vi "Result.Test Result to Factory Logix Xlink Adapter.vi"(5 "Overall Result Only":bool, 6 "Prefixes":T1={"Test Run"="TestRun.", "Client Setup"="StaSetup.", "Client SW"="StaSW.", "Client HW"="StaHW.", "Attribute"="Str.", "Numeric"="Num.", "Client ID"="Sta."}, 7 "Remove Headings":bool, 8 "error in":errorcluster, 9 "Add Prefixes":bool, 10 "Test Result":T2={"#attributes"={"Version"="MTE_1.0.0"}, "Station"={"Name"="", "PN"="", "SN"="", "Rev"="", "PC Name"="", "Location"="", "HW_Config"={"HW_Item"=[]}, "SW_Config"={"SW_Item"=[]}}, "Test Run"={"Operator"="", "Start Time"=timestamp(0 s since 1904-01-01), "Duration(s)"=0.0, "Mode"="", "Comment"="", "ProcessStep"=""}, "Test Sequence"={"Name"="", "Config"={"Config_Item"=[]}}, "UUTs"={"UUT"=[]}} {"UUTs"."UUT"."Measurements"."Measurement"."Status" items=["LOG", "PASS", "FAIL", "ERROR"]}, 11 "Path":path) -> (0 "error out":errorcluster)   [LabVIEW 2018]
uses:
  TestResult.FullResultData.ctl
  TestResult.Station Info.ctl
  TestResult.HW Item.ctl
  TestResult.SW Item.ctl
  TestResult.Test Run Info.ctl
  TestResult.Test Info.ctl
  TestResult.UUT Result.ctl
  TestResult.Symptom.ctl
  TestResult.Symptom.State.ctl
  Result.Measurement Item.ctl
  Result.Measurement and Attribute Item Status.ctl
  TestResult.UUTInfo.ctl
  Result.Factory Logix XLink Adapter, Data Prefixes.ctl
  Result.Factory Logix XLink Adapter, Measurement Item.ctl
  Result.Factory Logix XLink Adapter.ctl
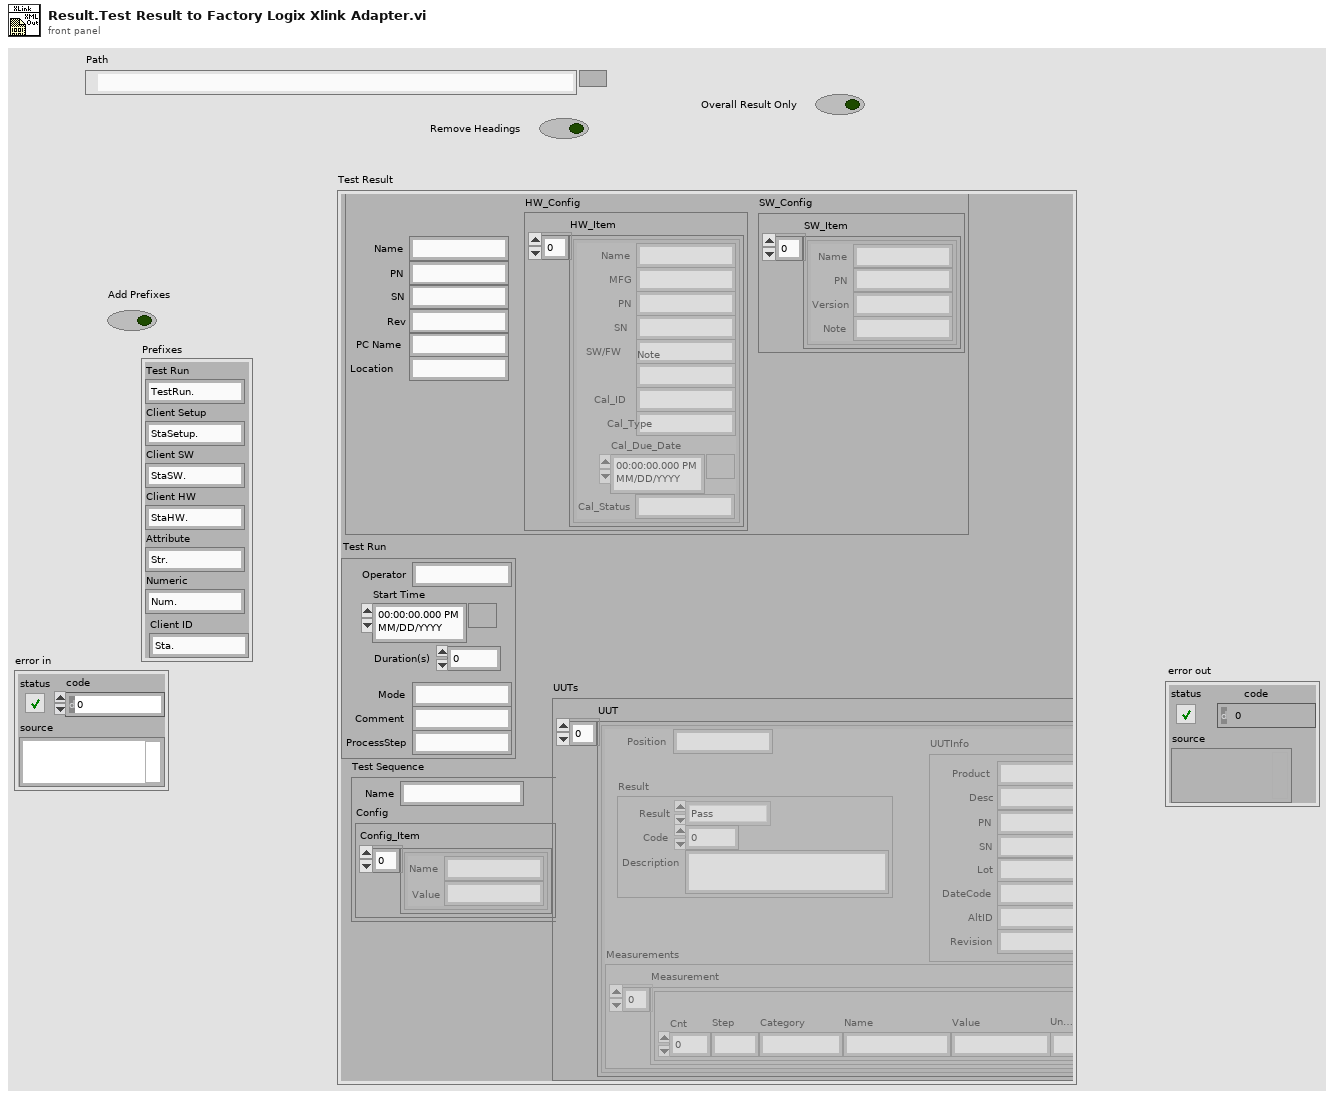
[diagram p1: front panel]
types:
  T1 = typedef "Result.Factory Logix XLink Adapter, Data Prefixes.ctl" = cluster{"Test Run":string, "Client Setup":string, "Client SW":string, "Client HW":string, "Attribute":string, "Numeric":string, "Client ID":string}
  T2 = typedef "TestResult.FullResultData.ctl" = cluster{"#attributes":cluster{"Version":string}, "Station":T3, "Test Run":T6, "Test Sequence":T7, "UUTs":cluster{"UUT":T8[]}}
  T3 = typedef "TestResult.Station Info.ctl" = cluster{"Name":string, "PN":string, "SN":string, "Rev":string, "PC Name":string, "Location":string, "HW_Config":cluster{"HW_Item":T4[]}, "SW_Config":cluster{"SW_Item":T5[]}}
  T4 = typedef "TestResult.HW Item.ctl" = cluster{"Name":string, "MFG":string, "PN":string, "SN":string, "SW/FW":string, "Note":string, "Cal_ID":string, "Cal_Type":string, "Cal_Due_Date":timestamp, "Cal_Status":string}
  T5 = typedef "TestResult.SW Item.ctl" = cluster{"Name":string, "PN":string, "Version":string, "Note":string}
  T6 = typedef "TestResult.Test Run Info.ctl" = cluster{"Operator":string, "Start Time":timestamp, "Duration(s)":dbl, "Mode":string, "Comment":string, "ProcessStep":string}
  T7 = typedef "TestResult.Test Info.ctl" = cluster{"Name":string, "Config":cluster{"Config_Item":cluster{"Name":string, "Value":string}[]}}
  T8 = typedef "TestResult.UUT Result.ctl" = cluster{"Position":string, "Result":T9, "Measurements":cluster{"Measurement":T11[]}, "UUTInfo":T13}
  T9 = typedef "TestResult.Symptom.ctl" = cluster{"Result":T10, "Code":i32, "Description":string}
  T10 = typedef "TestResult.Symptom.State.ctl" = enum16{"Pass", "Fail", "Error", "Aborted", "Completed", "Logged"}
  T11 = typedef "Result.Measurement Item.ctl" = cluster{"Cnt":i32, "Step":string, "Category":string, "Name":string, "Value":string, "Units":string, "LimType":string, "LL":string, "UL":string, "Status":T12, "Code":i32, "Desc":string, "Time":timestamp}
  T12 = typedef "Result.Measurement and Attribute Item Status.ctl" = i32
  T13 = typedef "TestResult.UUTInfo.ctl" = cluster{"Product":string, "Desc":string, "PN":string, "SN":string, "Lot":string, "DateCode":string, "AltID":string, "Revision":string, "Properties":cluster{"Property":cluster{"Name":string, "Value":string}[]}}
  T14 = typedef "Result.Factory Logix XLink Adapter, Measurement Item.ctl" = cluster{"Name":string, "Sequence":i32, "Measurement Type":string, "Result":string, "Value":string, "Units":string, "Nominal":string, "LowerLimit":string, "UpperLimit":string, "FailDesc":string, "DateAndTime":string}
  T15 = typedef "Result.Factory Logix XLink Adapter.ctl" = cluster{"Operator":string, "ParentBarcode":string, "Measurements":cluster{"Measurement":T14[]}}
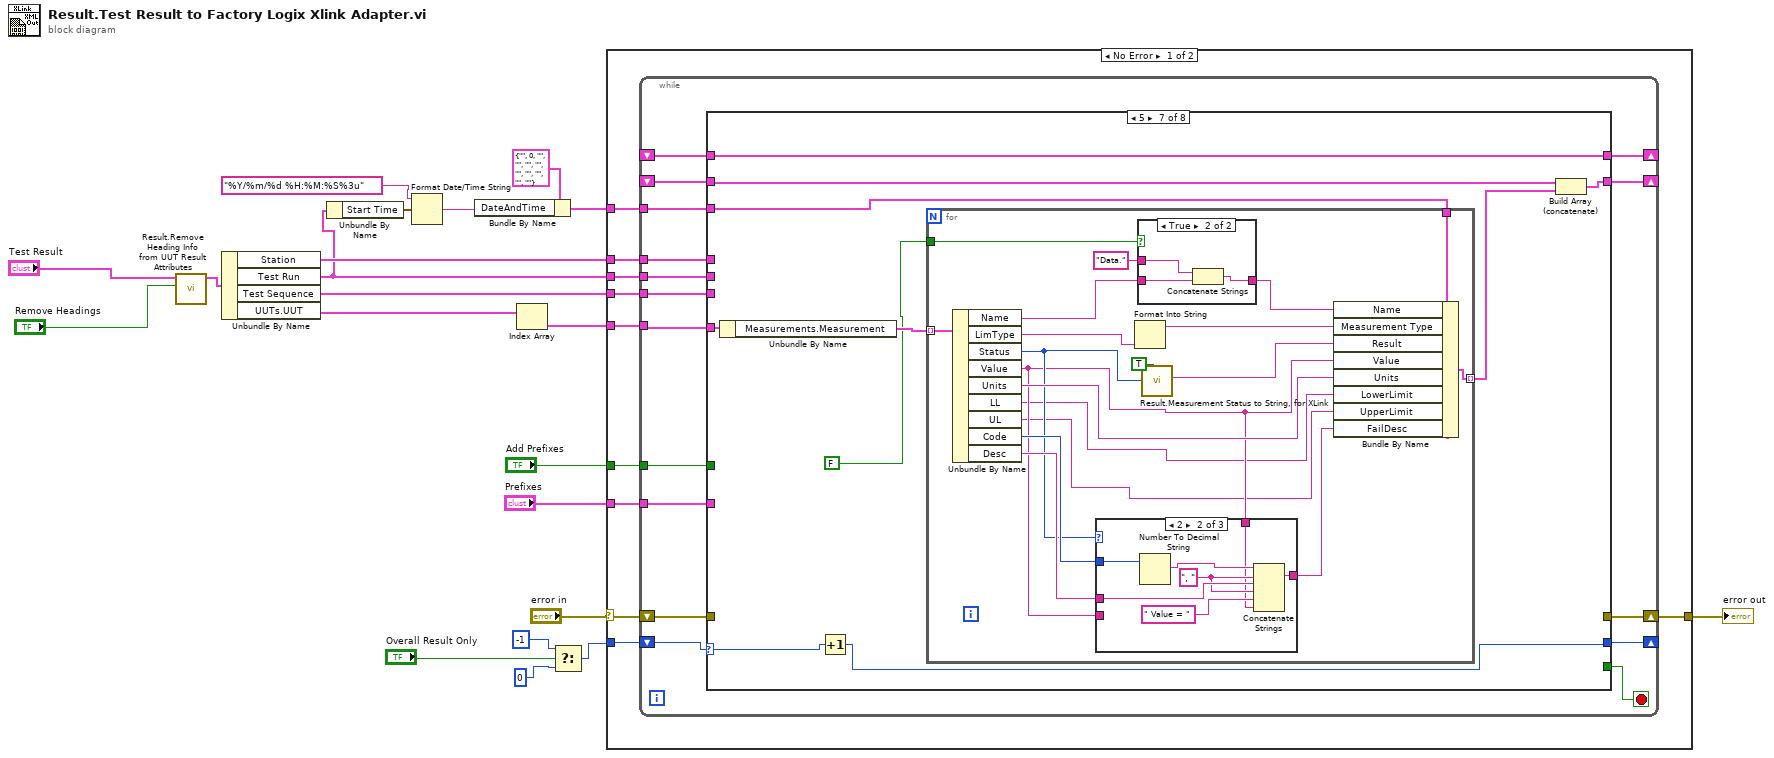
[diagram p0: block diagram]
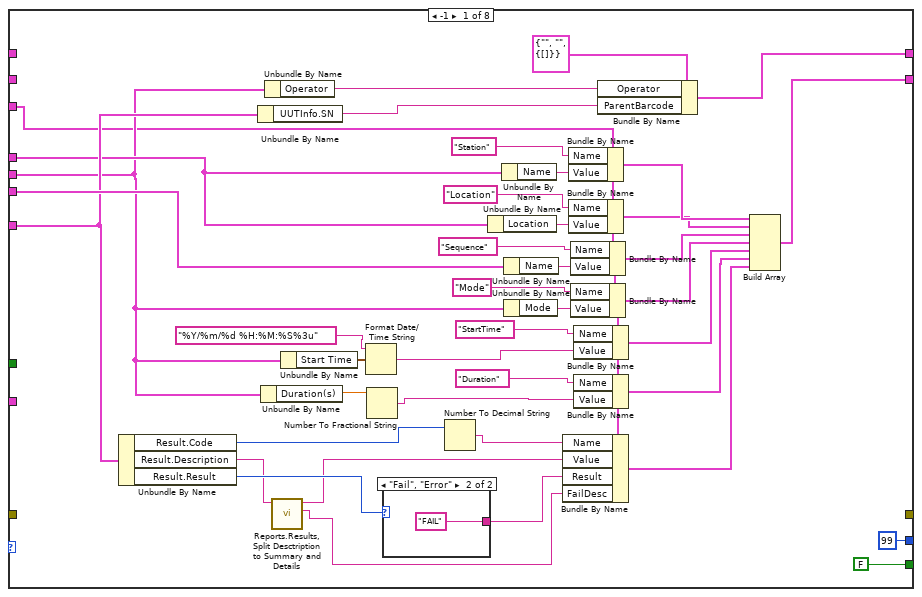
[diagram p2: hidden frame]
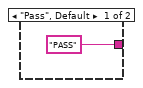
[diagram p3: hidden frame]
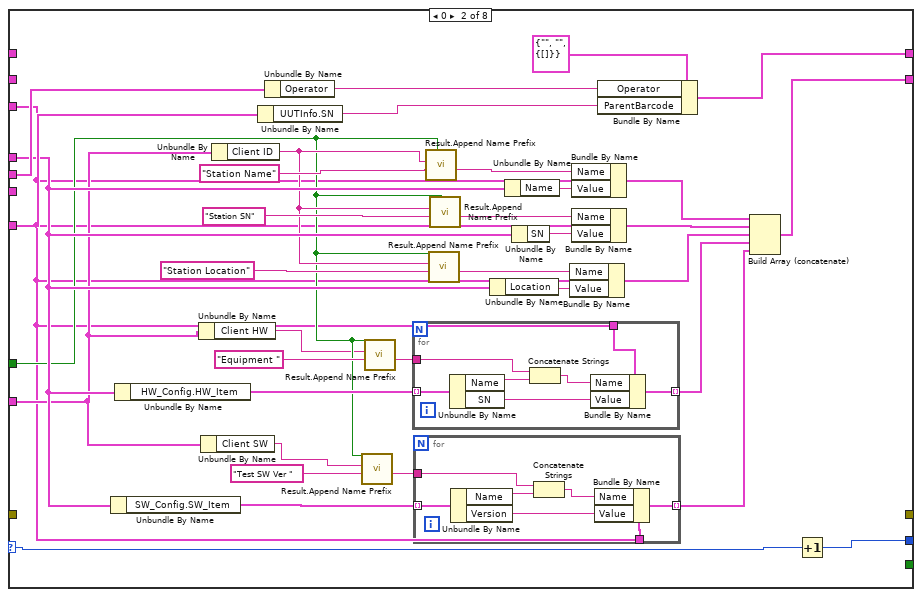
[diagram p4: hidden frame]
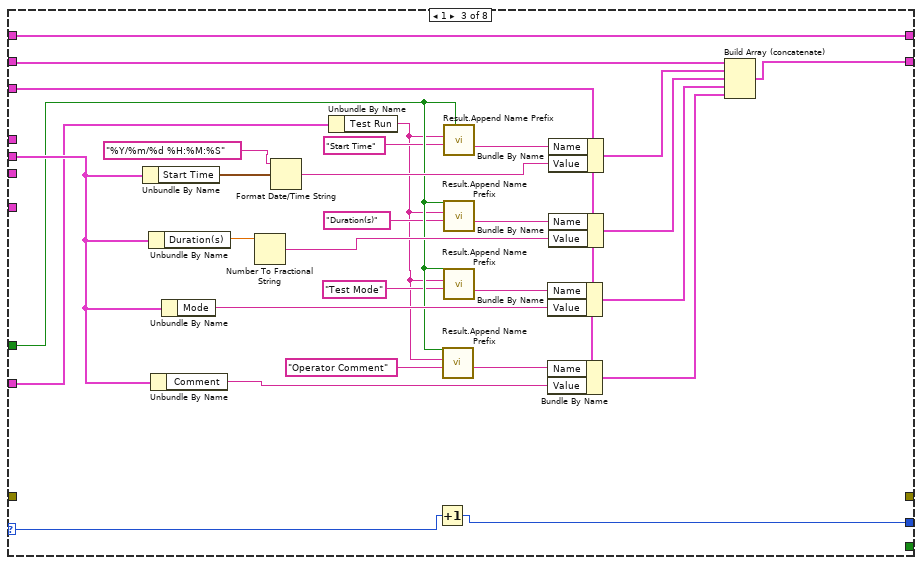
[diagram p5: hidden frame]
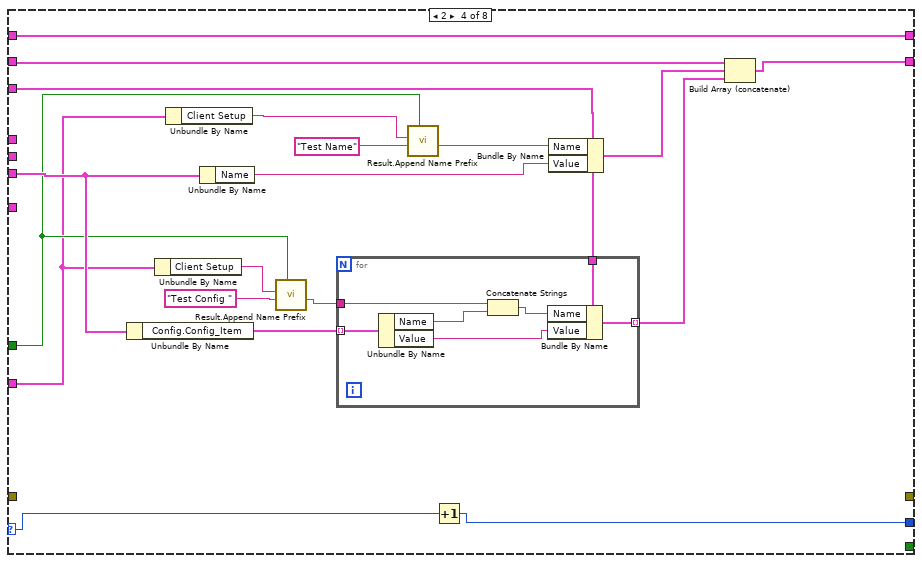
[diagram p6: hidden frame]
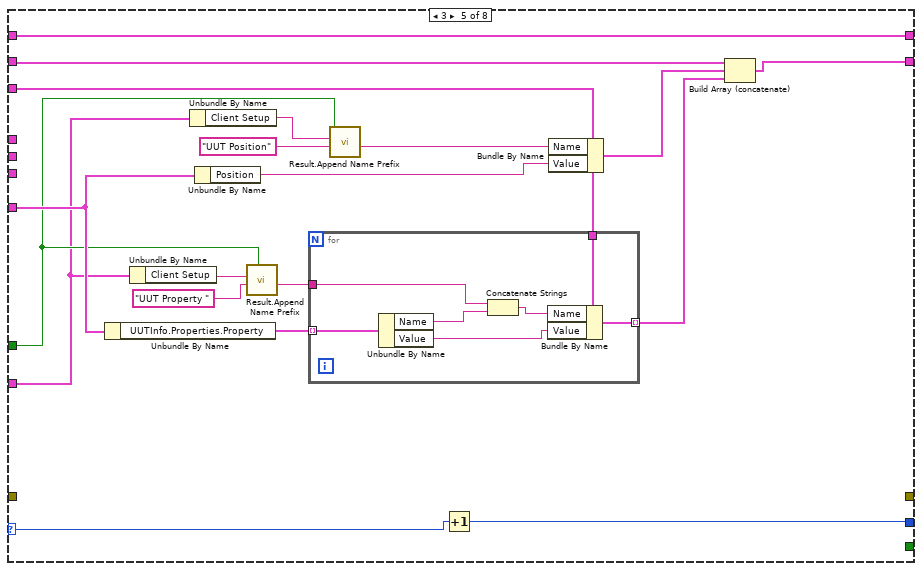
[diagram p7: hidden frame]
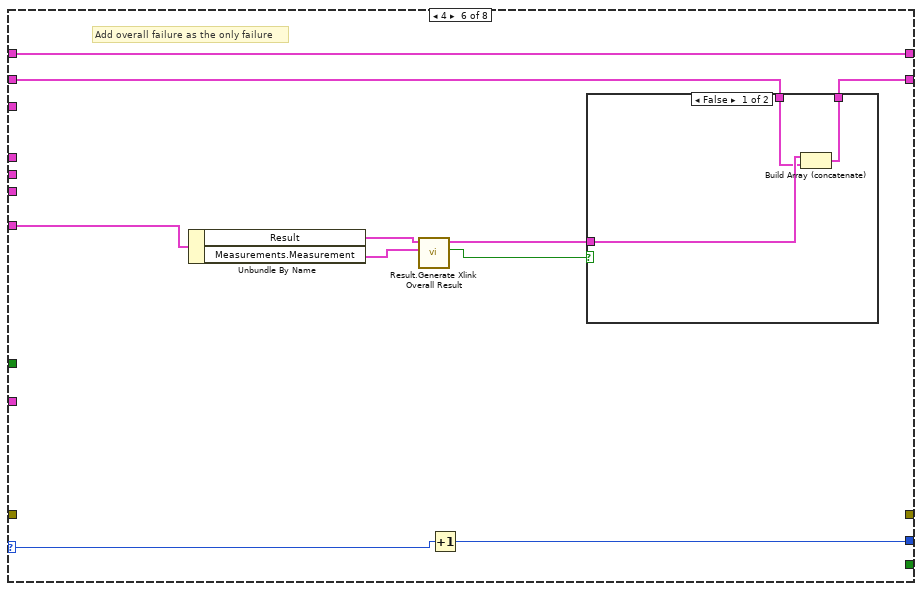
[diagram p8: hidden frame]
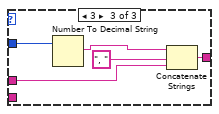
[diagram p12: hidden frame]
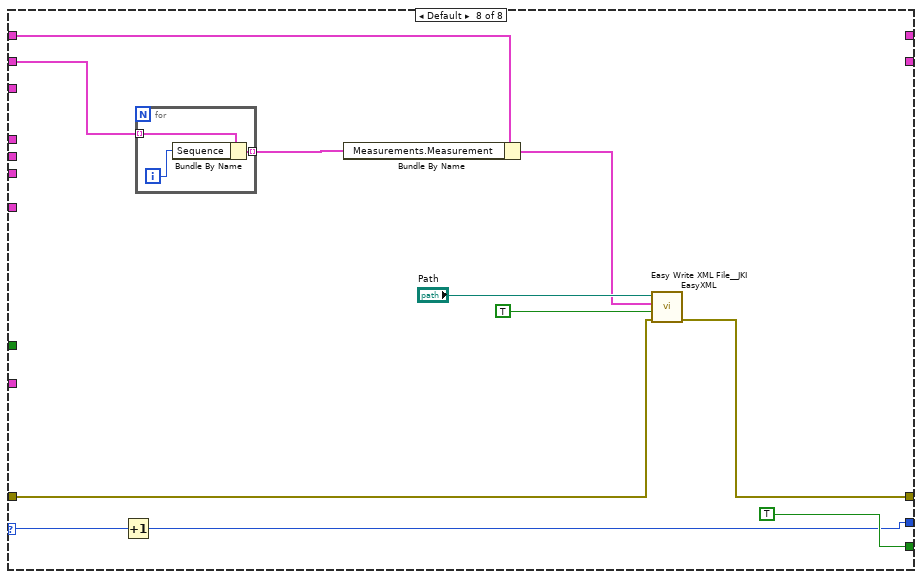
[diagram p13: hidden frame]
diagram:
  n1 = call "Result.Remove Heading Info from UUT Result Attributes.vi"("Remove Headings"="Remove Headings", "Data"="Test Result") -> ("Data Out"=w14:T2)  [unwired: 9 in]
  n2 = Unbundle By Name(w14) -> ("Station"=w17:T3, "Test Run"=w6:T6, "Test Sequence"=w16:T7, "UUTs.UUT"=w19:T8[])
  n3 = Unbundle By Name(w6) -> ("Start Time"=w7:timestamp)
  n4 = Format Date/Time String(time format string (%c)="%Y/%m/%d %H:%M:%S%3u", seconds (now)=w7) -> (date/time string=w5:string)  [unwired: 1 in]
  n5 = Bundle By Name(cluster=T14 {"Name"="", "Sequence"=0, "Measurement Type"="", "Result"="", "Value"="", "Units"="", "Nominal"="", "LowerLimit"="", "UpperLimit"="", "FailDesc"="", "DateAndTime"=""} ("Measurement"), "DateAndTime"=w5) -> (w9:T14)
  n6 = Index Array(array=w19) -> (element=w18:T8)  [unwired: 1 in]
  n7 = Select(t=-1, s="Overall Result Only", f=0) -> (s? t:f=w1:i32)
  n8 = case shown="No Error" "error in" {
    selector: "error in" -> [w30 w295]
    tunnel: [w31 w295] -> w21
    tunnel: w18 -> [w29 _]
    tunnel: w17 -> [w28 _]
    tunnel: w6 -> [w27 _]
    tunnel: w16 -> [w26 _]
    tunnel: "Prefixes" -> [w25 _]
    tunnel: "Add Prefixes" -> [w24 _]
    tunnel: w9 -> [w23 _]
    tunnel: w1 -> [w22 _]
    frame No Error {
      n9 = while {
        shift-right: [w47] -> w31
        shift-left: w30 -> [w46]
        shift-right: [w44] -> _
        shift-left: _ -> [w45]
        tunnel: w29 -> [w42]
        tunnel: w28 -> [w40]
        tunnel: w27 -> [w43]
        tunnel: w26 -> [w39]
        shift-right: [w41] -> _
        shift-left: _ -> [w37]
        tunnel: w25 -> [w36]
        tunnel: w24 -> [w35]
        tunnel: w23 -> [w34]
        shift-right: [w32] -> _
        shift-left: w22 -> [w33]
        stop <- w38 stop-if-true
        n10 = case shown="5" w33 {
          selector: w33 -> [_ w91 w142 w171 w197 w223 w237 w282]
          tunnel: [_ _ _ _ _ _ _ w290] -> w47
          tunnel: w46 -> [_ _ _ _ _ _ _ w288]
          tunnel: w45 -> [_ _ w169 w188 w214 w231 w245 w287]
          tunnel: [w87 w125 w169 w188 w214 w231 w245 _] -> w44
          tunnel: w43 -> [w55 w124 w162 _ _ _ _ _]
          tunnel: w42 -> [w74 w123 _ _ w207 w228 w241 _]
          tunnel: [w83 w119 w166 w185 w211 w229 w240 _] -> w41
          tunnel: w37 -> [_ _ w168 w187 w213 w230 w244 w286]
          tunnel: w40 -> [w66 w109 _ _ _ _ _ _]
          tunnel: w39 -> [w75 _ _ w184 _ _ _ _]
          tunnel: [FALSE _ _ _ _ _ _ TRUE] -> w38
          tunnel: w36 -> [_ w96 w145 w174 w199 _ _ _]
          tunnel: w35 -> [_ w97 w154 w176 w202 _ _ _]
          tunnel: w34 -> [w53 w93 w143 w172 w198 _ w238 _]
          tunnel: [99 w92 w141 w170 w196 w222 w236 w281] -> w32
          frame -1 {
            n11 = Unbundle By Name(w74) -> ("Result.Code"=w73:i32, "Result.Description"=w50:string, "Result.Result"=w71:T10)
            n12 = Unbundle By Name(w74) -> ("UUTInfo.SN"=w86:string)
            n13 = Unbundle By Name(w55) -> ("Duration(s)"=w56:dbl)
            n14 = Unbundle By Name(w55) -> ("Operator"=w85:string)
            n15 = call "Reports.Results, Split Desctription to Summary and Details.vi"("Description"=w50) -> ("Details"=w48:string, "Summary Description"=w49:string)  [unwired: 9 in]
            n16 = Unbundle By Name(w55) -> ("Start Time"=w59:timestamp)
            n17 = Format Date/Time String(time format string (%c)="%Y/%m/%d %H:%M:%S%3u", seconds (now)=w59) -> (date/time string=w57:string)  [unwired: 1 in]
            n18 = Number To Fractional String(number=w56) -> (F-format string=w54:string)  [unwired: 3 in]
            n19 = case shown="\"Fail\", \"Error\"" w71 {
              tunnel: ["PASS" "FAIL"] -> w70
              frame "Pass", Default {
              }
              frame "Fail", "Error" {
              }
            }
            n20 = Number To Decimal String(number=w73) -> (decimal integer string=w72:string)  [unwired: 1 in]
            n21 = Unbundle By Name(w66) -> ("Location"=w67:string)
            n22 = Unbundle By Name(w66) -> ("Name"=w82:string)
            n23 = Unbundle By Name(w75) -> ("Name"=w80:string)
            n24 = Unbundle By Name(w55) -> ("Mode"=w77:string)
            n25 = Bundle By Name(cluster=w53, "Name"=w72, "Value"=w49, "Result"=w70, "FailDesc"=w48) -> (w52:T14)
            n26 = Bundle By Name(cluster=w53, "Name"="Station", "Value"=w82) -> (w84:T14)
            n27 = Bundle By Name(cluster=w53, "Name"="Location", "Value"=w67) -> (w65:T14)
            n28 = Bundle By Name(cluster=w53, "Name"="Sequence", "Value"=w80) -> (w79:T14)
            n29 = Bundle By Name(cluster=w53, "Name"="Mode", "Value"=w77) -> (w69:T14)
            n30 = Bundle By Name(cluster=w53, "Name"="StartTime", "Value"=w57) -> (w61:T14)
            n31 = Bundle By Name(cluster=w53, "Name"="Duration", "Value"=w54) -> (w51:T14)
            n32 = Bundle By Name(cluster=T15 {"Operator"="", "ParentBarcode"="", "Measurements"={"Measurement"=[]}} ("TestData"), "Operator"=w85, "ParentBarcode"=w86) -> (w87:T15)
            n33 = Build Array(w84, w65, w79, w69, w61, w51, w52) -> (w83:T14[])
          }
          frame 0 {
            n34 = Unbundle By Name(w109) -> ("SW_Config.SW_Item"=w111:T5[])
            n35 = Unbundle By Name(w109) -> ("HW_Config.HW_Item"=w113:T4[])
            n36 = Unbundle By Name(w96) -> ("Client HW"=w95:string)
            n37 = Unbundle By Name(w96) -> ("Client SW"=w94:string)
            n38 = Unbundle By Name(w96) -> ("Client ID"=w104:string)
            n39 = Unbundle By Name(w123) -> ("UUTInfo.SN"=w122:string)
            n40 = Unbundle By Name(w124) -> ("Operator"=w121:string)
            n41 = call "Result.Append Name Prefix.vi"("Append"=w97, "Name"="Test SW Ver ", "Prefix"=w94) -> ("Name Out"=w99:string)  [unwired: 8 in]
            n42 = call "Result.Append Name Prefix.vi"("Append"=w97, "Name"="Equipment ", "Prefix"=w95) -> ("Name Out"=w101:string)  [unwired: 8 in]
            n43 = for {
              tunnel: w113 -> [w140] mode=indexing
              tunnel: [w138] -> w112 mode=indexing
              tunnel: w101 -> [w135]
              tunnel: w93 -> [w134]
              n44 = Unbundle By Name(w140) -> ("Name"=w137:string, "SN"=w139:string)
              n45 = Concatenate Strings(w135, w137) -> (w136:string)
              n46 = Bundle By Name(cluster=w134, "Name"=w136, "Value"=w139) -> (w138:T14)
            }
            n47 = for {
              tunnel: w111 -> [w133] mode=indexing
              tunnel: [w131] -> w110 mode=indexing
              tunnel: w99 -> [w128]
              tunnel: w93 -> [w127]
              n48 = Unbundle By Name(w133) -> ("Name"=w130:string, "Version"=w132:string)
              n49 = Concatenate Strings(w128, w130) -> (w129:string)
              n50 = Bundle By Name(cluster=w127, "Name"=w129, "Value"=w132) -> (w131:T14)
            }
            n51 = call "Result.Append Name Prefix.vi"("Append"=w97, "Name"="Station Name", "Prefix"=w104) -> ("Name Out"=w107:string)  [unwired: 8 in]
            n52 = call "Result.Append Name Prefix.vi"("Append"=w97, "Name"="Station Location", "Prefix"=w104) -> ("Name Out"=w102:string)  [unwired: 8 in]
            n53 = call "Result.Append Name Prefix.vi"("Append"=w97, "Name"="Station SN", "Prefix"=w104) -> ("Name Out"=w106:string)  [unwired: 8 in]
            n54 = Unbundle By Name(w109) -> ("Location"=w116:string)
            n55 = Unbundle By Name(w109) -> ("Name"=w118:string)
            n56 = Unbundle By Name(w109) -> ("SN"=w117:string)
            n57 = Bundle By Name(cluster=w93, "Name"=w102, "Value"=w116) -> (w114:T14)
            n58 = Bundle By Name(cluster=w93, "Name"=w107, "Value"=w118) -> (w120:T14)
            n59 = Bundle By Name(cluster=w93, "Name"=w106, "Value"=w117) -> (w115:T14)
            n60 = Bundle By Name(cluster=T15 {"Operator"="", "ParentBarcode"="", "Measurements"={"Measurement"=[]}} ("TestData"), "Operator"=w121, "ParentBarcode"=w122) -> (w125:T15)
            n61 = Build Array (concatenate)(w120, w115, w114, w112, w110) -> (w119:T14[])
            n62 = Increment(x=w91) -> (x+1=w92:i32)
          }
          frame 1 {
            n63 = Unbundle By Name(w162) -> ("Start Time"=w165:timestamp)
            n64 = Unbundle By Name(w162) -> ("Duration(s)"=w161:dbl)
            n65 = Unbundle By Name(w162) -> ("Comment"=w158:string)
            n66 = Unbundle By Name(w162) -> ("Mode"=w159:string)
            n67 = Number To Fractional String(number=w161) -> (F-format string=w160:string)  [unwired: 3 in]
            n68 = Format Date/Time String(time format string (%c)="%Y/%m/%d %H:%M:%S", seconds (now)=w165) -> (date/time string=w163:string)  [unwired: 1 in]
            n69 = Unbundle By Name(w145) -> ("Test Run"=w144:string)
            n70 = Increment(x=w142) -> (x+1=w141:i32)
            n71 = call "Result.Append Name Prefix.vi"("Append"=w154, "Name"="Operator Comment", "Prefix"=w144) -> ("Name Out"=w152:string)  [unwired: 8 in]
            n72 = call "Result.Append Name Prefix.vi"("Append"=w154, "Name"="Start Time", "Prefix"=w144) -> ("Name Out"=w147:string)  [unwired: 8 in]
            n73 = call "Result.Append Name Prefix.vi"("Append"=w154, "Name"="Duration(s)", "Prefix"=w144) -> ("Name Out"=w149:string)  [unwired: 8 in]
            n74 = call "Result.Append Name Prefix.vi"("Append"=w154, "Name"="Test Mode", "Prefix"=w144) -> ("Name Out"=w151:string)  [unwired: 8 in]
            n75 = Bundle By Name(cluster=w143, "Name"=w151, "Value"=w159) -> (w156:T14)
            n76 = Bundle By Name(cluster=w143, "Name"=w152, "Value"=w158) -> (w155:T14)
            n77 = Bundle By Name(cluster=w143, "Name"=w147, "Value"=w163) -> (w167:T14)
            n78 = Bundle By Name(cluster=w143, "Name"=w149, "Value"=w160) -> (w157:T14)
            n79 = Build Array (concatenate)(w168, w167, w157, w156, w155) -> (w166:T14[])
          }
          frame 2 {
            n80 = Unbundle By Name(w184) -> ("Config.Config_Item"=w182:cluster{"Name":string, "Value":string}[])
            n81 = Unbundle By Name(w174) -> ("Client Setup"=w175:string)
            n82 = Unbundle By Name(w174) -> ("Client Setup"=w173:string)
            n83 = Unbundle By Name(w184) -> ("Name"=w183:string)
            n84 = call "Result.Append Name Prefix.vi"("Append"=w176, "Name"="Test Config ", "Prefix"=w175) -> ("Name Out"=w177:string)  [unwired: 8 in]
            n85 = for {
              tunnel: w182 -> [w194] mode=indexing
              tunnel: [w191] -> w181 mode=indexing
              tunnel: w172 -> [w190]
              tunnel: w177 -> [w189]
              n86 = Unbundle By Name(w194) -> ("Name"=w193:string, "Value"=w192:string)
              n87 = Concatenate Strings(w189, w193) -> (w195:string)
              n88 = Bundle By Name(cluster=w190, "Name"=w195, "Value"=w192) -> (w191:T14)
            }
            n89 = call "Result.Append Name Prefix.vi"("Append"=w176, "Name"="Test Name", "Prefix"=w173) -> ("Name Out"=w179:string)  [unwired: 8 in]
            n90 = Increment(x=w171) -> (x+1=w170:i32)
            n91 = Bundle By Name(cluster=w172, "Name"=w179, "Value"=w183) -> (w186:T14)
            n92 = Build Array (concatenate)(w187, w186, w181) -> (w185:T14[])
          }
          frame 3 {
            n93 = Unbundle By Name(w207) -> ("UUTInfo.Properties.Property"=w209:cluster{"Name":string, "Value":string}[])
            n94 = Unbundle By Name(w199) -> ("Client Setup"=w203:string)
            n95 = Unbundle By Name(w199) -> ("Client Setup"=w205:string)
            n96 = Unbundle By Name(w207) -> ("Position"=w210:string)
            n97 = call "Result.Append Name Prefix.vi"("Append"=w202, "Name"="UUT Property ", "Prefix"=w203) -> ("Name Out"=w200:string)  [unwired: 8 in]
            n98 = for {
              tunnel: w209 -> [w220] mode=indexing
              tunnel: [w217] -> w208 mode=indexing
              tunnel: w198 -> [w216]
              tunnel: w200 -> [w215]
              n99 = Unbundle By Name(w220) -> ("Name"=w219:string, "Value"=w218:string)
              n100 = Concatenate Strings(w215, w219) -> (w221:string)
              n101 = Bundle By Name(cluster=w216, "Name"=w221, "Value"=w218) -> (w217:T14)
            }
            n102 = call "Result.Append Name Prefix.vi"("Append"=w202, "Name"="UUT Position", "Prefix"=w205) -> ("Name Out"=w204:string)  [unwired: 8 in]
            n103 = Increment(x=w197) -> (x+1=w196:i32)
            n104 = Bundle By Name(cluster=w198, "Name"=w204, "Value"=w210) -> (w212:T14)
            n105 = Build Array (concatenate)(w213, w212, w208) -> (w211:T14[])
          }
          frame 4 {
            # "Add overall failure as the only failure"
            n106 = Unbundle By Name(w228) -> ("Result"=w227:T9, "Measurements.Measurement"=w226:T11[])
            n107 = call "Result.Generate Xlink Overall Result.vi"("Measurements"=w226, "Result"=w227) -> ("PASS"=w225:bool, "Measurement"=w224:T14)  [unwired: 8 in]
            n108 = Increment(x=w223) -> (x+1=w222:i32)
            n109 = case shown="False" w225 {
              tunnel: w230 -> [w232 w235]
              tunnel: [w234 w235] -> w229
              tunnel: w224 -> [w233 _]
              frame False {
                n110 = Build Array (concatenate)(w233, w232) -> (w234:T14[])
              }
              frame True {
              }
            }
          }
          frame 5 {
            n111 = Unbundle By Name(w241) -> ("Measurements.Measurement"=w243:T11[])
            n112 = Increment(x=w237) -> (x+1=w236:i32)
            n113 = for {
              tunnel: w243 -> [w264] mode=indexing
              tunnel: [w263] -> w242 mode=indexing
              tunnel: FALSE -> [w251]
              tunnel: w238 -> [w250]
              n114 = Unbundle By Name(w264) -> ("Name"=w253:string, "LimType"=w262:string, "Status"=w255:T12, "Value"=w249:string, "Units"=w260:string, "LL"=w248:string, "UL"=w247:string, "Code"=w259:i32, "Desc"=w258:string)
              n115 = case shown="2" w255 {
                tunnel: w259 -> [_ w275 w276]
                tunnel: w258 -> [_ w272 w277]
                tunnel: [_ w273 w278] -> w257
                tunnel: w249 -> [_ _ _]
                tunnel: w249 -> [_ w269 _]
                frame 0, Default {
                }
                frame 2 {
                  w271 = ", "
                  n116 = Number To Decimal String(number=w275) -> (decimal integer string=w274:string)  [unwired: 1 in]
                  n117 = Concatenate Strings(w274, w271, w272, w271, " Value = ", w269) -> (w273:string)
                }
                frame 3 {
                  n118 = Number To Decimal String(number=w276) -> (decimal integer string=w280:string)  [unwired: 1 in]
                  n119 = Concatenate Strings(w280, ", ", w277) -> (w278:string)
                }
              }
              n120 = Format Into String(w262) -> (resulting string=w261:string)  [unwired: 3 in, 1 out]
              n121 = case shown="True" w251 {
                tunnel: w253 -> [w265 w268]
                tunnel: [w265 w266] -> w252
                tunnel: "Data." ("Numeric") -> [_ w267]
                frame False {
                }
                frame True {
                  n122 = Concatenate Strings(w267, w268) -> (w266:string)
                }
              }
              n123 = call "Result.Measurement Status to String, for XLink.vi"("Fail = OutOfTolerance"=TRUE, "Status"=w255) -> ("resulting string"=w256:string)  [unwired: 6 in]
              n124 = Bundle By Name(cluster=w250, "Name"=w252, "Measurement Type"=w261, "Result"=w256, "Value"=w249, "Units"=w260, "LowerLimit"=w248, "UpperLimit"=w247, "FailDesc"=w257) -> (w263:T14)
            }
            n125 = Build Array (concatenate)(w244, w242) -> (w240:T14[])
          }
          frame Default {
            n126 = Increment(x=w282) -> (x+1=w281:i32)
            n127 = for {
              tunnel: w286 -> [w294] mode=indexing
              tunnel: [w292] -> w285 mode=indexing
              i -> [w293]
              n128 = Bundle By Name(cluster=w294, "Sequence"=w293) -> (w292:T14)
            }
            n129 = Bundle By Name(cluster=w287, "Measurements.Measurement"=w285) -> (w284:T15)
            n130 = call <vilib>:"Easy Write XML File__JKI EasyXML.vi"("error in (no error)"=w288, "Overwrite File? (false)"=TRUE, "LabVIEW Data"=w284, "XML File Path"="Path") -> ("error out"=w290:errorcluster)  [unwired: 6 in, 1 out]
          }
        }
      }
    }
    frame Error {
    }
  }
  "error out" <- w21
